vi "PCO_GetFlimRelativePhase.vi"(8 "error in (no error)":errorcluster {"code" format="%x"}, 11 "ph":u64) -> (0 "error out":errorcluster {"code" format="%x"}, 1 "dwPhaseMilliDeg":u32, 2 "ErrorMessage":i32 format="%x", 3 "ph out":u64)   [LabVIEW 2020, in "SDK.lvlib" / "SpecialCommandsFlim.lvlib"]
doc: "<b>Description:</b>\nThis function can be used to query the current relative phase setting, which is used when the camera is configured for manual phase shifting.\nSee function PCO_SetFlimPhaseSequenceParameter.\n\n<b>Supported camera type:</b>\npco.flim\n\n<b>Descriptor dependency:</b>\nNone"
uses:
  SpecialCommandsFlim.lvlib
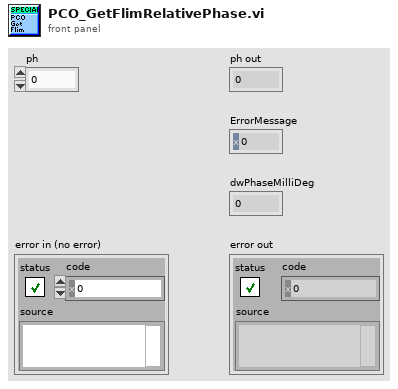
[diagram p1: front panel]
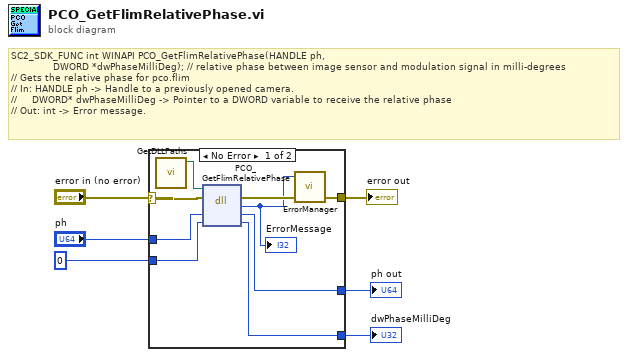
[diagram p0: block diagram]
diagram:
  # "SC2_SDK_FUNC int WINAPI PCO_GetFlimRelativePhase(HANDLE ph, \n              DWORD *dwPhaseMilliDeg); // relative phase between image sensor and modulation signal in milli-degrees\n// Gets the relative phase for pco.flim\n// In: HANDLE ph -> Handle to a previously opened camera.\n//     DWORD* dwPhaseMilliDeg -> Pointer to a DWORD variable to receive the relative phase\n// Out: int -> Error message."
  n1 = case shown="No Error" "error in (no error)" {
    selector: "error in (no error)" -> [w11 w18]
    tunnel: "ph" -> [w15 w17]
    tunnel: [w14 w17] -> w5
    tunnel: u32 0 ("dwPhaseMilliDeg") -> [w13 w16]
    tunnel: [w12 w16] -> w3
    tunnel: [w10 w18] -> w2
    frame No Error {
      n2 = call "GetDLLPaths.vi"() -> ("SC2_Cam_Path"=w7:path)  [unwired: 9 in, 2 out]
      n3 = dll-call lib="?" fn="PCO_GetFlimRelativePhase"(path in=w7, error in=w11, "ph"=w15, "dwPhaseMilliDeg"=w13) -> (error out=w9:errorcluster, "return type"=w8:i32, "ph"=w14:u64, "dwPhaseMilliDeg"=w12:u32)  [unwired: 1 in, 1 out]
      "ErrorMessage" <- w8
      n4 = call "ErrorManager.vi"("error in (no error)"=w9, "error code"=w8) -> ("error out"=w10:errorcluster)  [unwired: 3 in]
    }
    frame Error {
    }
  }
  "ph out" <- w5
  "dwPhaseMilliDeg" <- w3
  "error out" <- w2
